vi "ReadXMLAquatrakData.vi"() -> ()   [LabVIEW 2014]
panel:
  out "Mean":dbl format="%.3g"
  out "Std":dbl format="%.5g"
  in  "OK Button":bool
  in  "L":dbl
  in  "M":dbl
  in  "S":dbl
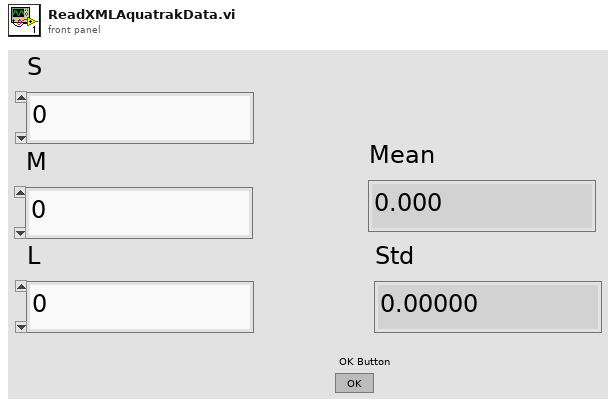
[diagram p1: front panel]
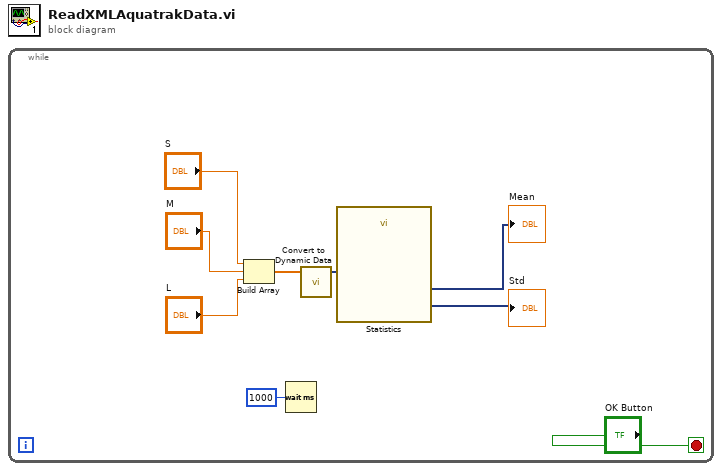
[diagram p0: block diagram]
diagram:
  n1 = while {
    stop <- "OK Button" stop-if-true
    n2 = Build Array("S", "M", "L") -> (w4:dbl[])
    n3 = Wait (ms)(milliseconds to wait=u32 1000) -> ()  [unwired: 1 out]
    n4 = call "Convert to Dynamic Data"("Array"=w4) -> ("Dynamic Data Type"=w3:dynamicdata)  [unwired: 3 in]
    n5 = call "Statistics"("Signals"=w3) -> ("Standard Dev"=→"Std":dynamicdata, "Arithmetic Mean"=→"Mean":dynamicdata)  [unwired: 24 in, 1 out]
  }
